vi "getPayloadRequirement.vi"(11 "SUBACK in":refnum<class "SUBACK.lvclass">) -> (2 "Requirement":T1, 3 "SUBACK out":refnum<class "SUBACK.lvclass">)   [LabVIEW 2013, in "SUBACK.lvclass"]
uses:
  SUBACK.lvclass
  ControlPacket/Requirement -- enum.ctl
  ControlPacket/ControlPacket.lvclass
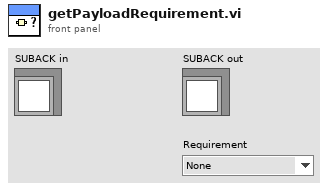
[diagram p1: front panel]
types:
  T1 = typedef "ControlPacket.lvclass/Requirement -- enum.ctl" = enum16{"None", "Optional", "Required"}
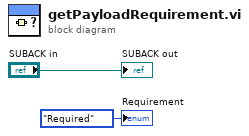
[diagram p0: block diagram]
diagram:
  "SUBACK out" <- "SUBACK in"
  "Requirement" <- Requirement_--_enum."Required" ("Requirement")
